vi "To 20 Bit.vi"(10 "index (0)":i32, 11 "array":u8[](array[numeric])) -> (3 "Result":u32)   [LabVIEW 2018, in "ColorSensor.lvlib"]
uses:
  ColorSensor.lvlib
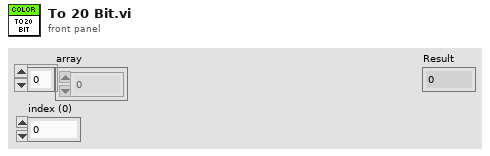
[diagram p1: front panel]
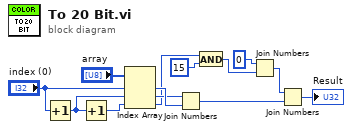
[diagram p0: block diagram]
diagram:
  n1 = Increment(x="index (0)") -> (x+1=w11:i32)
  n2 = Increment(x=w11) -> (x+1=w10:i32)
  n3 = Index Array(array="array", index #1="index (0)", index #2=w11, index #3=w10) -> (element #1=w9:u8, element #2=w8:u8, element #3=w3:u8)
  n4 = Join Numbers(hi=w8, lo=w9) -> ((hi.lo)=w6:u16)
  n5 = And(x=w3, y=u8 15) -> (x .and. y?=w2:u8)
  n6 = Join Numbers(hi=u8 0, lo=w2) -> ((hi.lo)=w5:u16)
  n7 = Join Numbers(hi=w5, lo=w6) -> ((hi.lo)=→"Result":u32)
